vi "Add New Service.vi"(8 "error in (no error)":errorcluster, 10 "Service Details":T1, 11 "Service Config Display in":refnum<class "Service Config Display.lvclass">) -> (0 "error out":errorcluster, 3 "Service Config Display out":refnum<class "Service Config Display.lvclass">)   [LabVIEW 2016, in "Assert Display.lvlib" / "Service Config Display.lvlib" / "Service Config Display.lvclass"]
uses:
  Service Config Display.lvclass
  C:/Program Files (x86)/National Instruments/LabVIEW 2016/vi.lib/ActorFramework/Actor/Actor.lvclass
  Service Details.ctl
  Assert Display/Assert Display/Item Configuration.ctl
  Items.ctl
  <vilib>/ActorFramework/Actor/Actor.lvclass/Actor.ctl
  Service Config Display.lvclass/Service Config Display.ctl
  Assert Display/Assert Display Messages/New Item Msg/New Item Msg.lvclass/New Item Msg.ctl
  <vilib>/ActorFramework/Message Enqueuer/Message Enqueuer.lvclass/Message Enqueuer.ctl
  <vilib>/ActorFramework/Message Enqueuer/Enqueue.vi
  Assert Display/Assert Display Messages/New Item Msg/New Item Msg.lvclass
  C:/Program Files (x86)/National Instruments/LabVIEW 2016/vi.lib/ActorFramework/Message/Message.lvclass
  <vilib>/ActorFramework/Message Priority Queue/Priority Enqueue.vi
  <vilib>/ActorFramework/Actor/Actor.lvclass
  Assert Display/Assert Display.lvlib
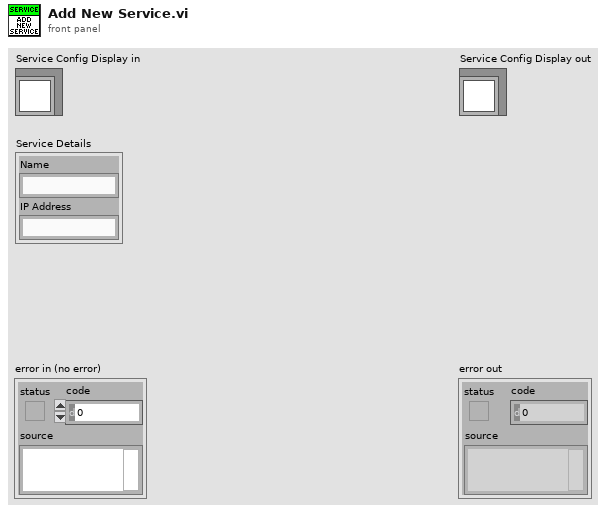
[diagram p1: front panel]
types:
  T1 = typedef "Assert Display.lvlib/Service Details.ctl" = cluster{"Name":string, "IP Address":string}
  T2 = typedef "Assert Display.lvlib/Items.ctl" = enum16{"Service", "Filter"}
  T3 = typedef "Assert Display.lvlib/Item Configuration.ctl" = cluster{"Item Type":T2, "Configuration":variant}
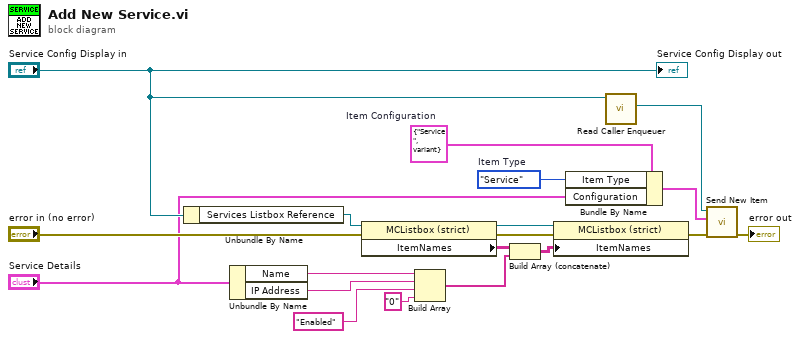
[diagram p0: block diagram]
diagram:
  w4 = Items."Service"  # Item Type
  w6 = T3 {"Item Type"=enum."Service", "Configuration"=variant}  # Item Configuration
  n1 = Unbundle By Name("Service Config Display in") -> ("Services Listbox Reference"=w19:refnum<vi>)
  n2 = Unbundle By Name("Service Details") -> ("Name"=w18:string, "IP Address"=w17:string)
  n3 = property class="MCListbox (strict)"(reference=w19, error in="error in (no error)") -> (reference out=w13:refnum<vi>, error out=w11:errorcluster, "ItemNames"=w15:string[][])
  n4 = Build Array(w18, w17, "Enabled" ("element"), "0" ("element")) -> (w16:string[])
  n5 = Build Array (concatenate)(w15, w16) -> (w14:string[][])
  n6 = property class="MCListbox (strict)"(reference=w13, error in=w11, "ItemNames"=w14) -> (error out=w2:errorcluster)  [unwired: 1 out]
  n7 = Bundle By Name(cluster=w6, "Item Type"=w4, "Configuration"="Service Details") -> (w5:T3)
  n8 = call <vilib>:"Read Caller Enqueuer.vi"("Actor"="Service Config Display in") -> ("Caller Enqueuer"=w7:refnum<class "Message Enqueuer.lvclass">)  [unwired: 10 in]
  n9 = call "Send New Item.vi"("error in (no error)"=w2, "Item Configuration"=w5, "Message Enqueuer"=w7) -> ("error out"=→"error out":errorcluster)  [unwired: 7 in, 1 out]
  "Service Config Display out" <- "Service Config Display in"
